vi "GenerateApriltagStandard41h12.vi"(8 "error in (no error)":errorcluster, 11 "ID":i32) -> (0 "error out":errorcluster, 3 "Tag Pixel Array":u8[][](array[numeric]) format="%.0x")   [LabVIEW 2020, in "feature_detection.lvlib"]
uses:
  feature_detection.lvlib
  TagIDOutOfRangeError.vi
  TagSetPixel.vi
  TagRotatePixelArray.vi
  <vilib>/Utility/error.llb/Error Cluster From Error Code.vi
  TagLayoutConvert.vi
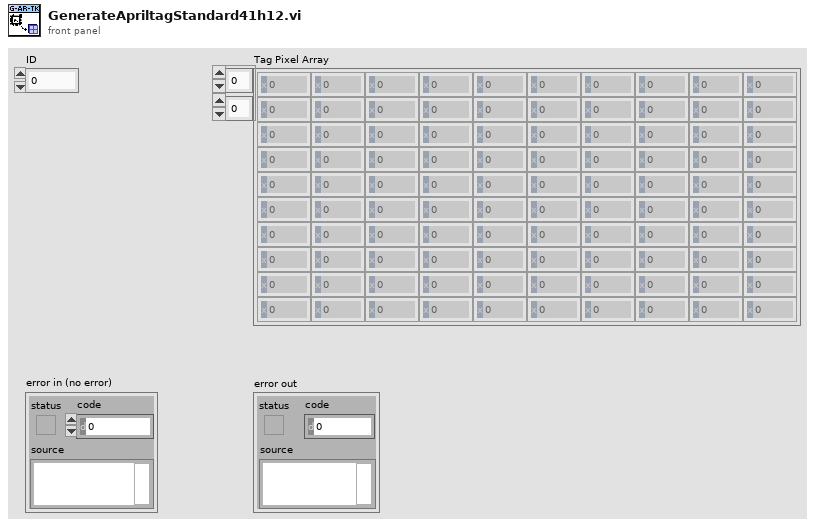
[diagram p1: front panel]
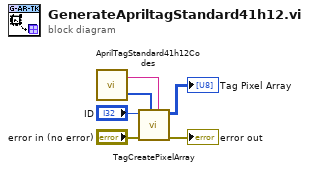
[diagram p0: block diagram]
diagram:
  n1 = call "AprilTagStandard41h12Codes.vi"() -> ("Codes"=w1:i64[], "Layout"=w2:string)  [unwired: 2 in]
  n2 = call "TagCreatePixelArray.vi"("Layout"=w2, "Codes"=w1, "error in (no error)"="error in (no error)", "ID"="ID") -> ("error out"=→"error out":errorcluster, "Pixels"=→"Tag Pixel Array":u8[][])  [unwired: 5 in, 1 out]
